vi "from string array.vi"(8 "error in (no error)":errorcluster, 9 "String Array":string[][](array[string]), 10 "version":string, 11 "PID Module configuration in":refnum<class "PID Module configuration.lvclass">) -> (0 "error out":errorcluster, 3 "PID Module configuration out":refnum<class "PID Module configuration.lvclass">)   [LabVIEW 2015, in "PID Module configuration.lvclass"]
uses:
  PID Module configuration.lvclass
  PID Module configuration.lvclass/PID Module configuration.ctl
  Write Lines.vi
  Get Line Name.vi
  <vilib>/NI/Tag Bus Module Framework/module configuration/FindDuplicate.vi
  <vilib>/Utility/error.llb/Error Cluster From Error Code.vi
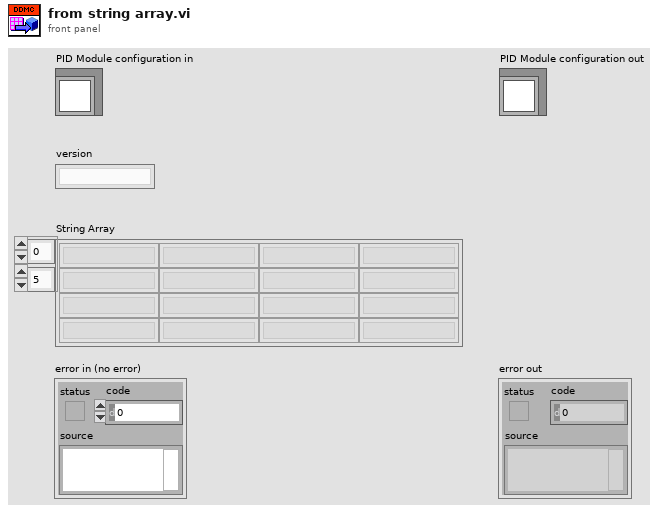
[diagram p1: front panel]
types:
  T1 = typedef "PID Module configuration.lvclass/Line.ctl" = cluster{"PID ID":string, "Setpoint":refnum<class "TBM channel.lvclass">, "Variable":refnum<class "TBM channel.lvclass">, "Output":refnum<class "TBM channel.lvclass">, "Output High":refnum<class "TBM channel.lvclass">, "Output Low":refnum<class "TBM channel.lvclass">, "P":refnum<class "TBM channel.lvclass">, "I":refnum<class "TBM channel.lvclass">, "D":refnum<class "TBM channel.lvclass">}
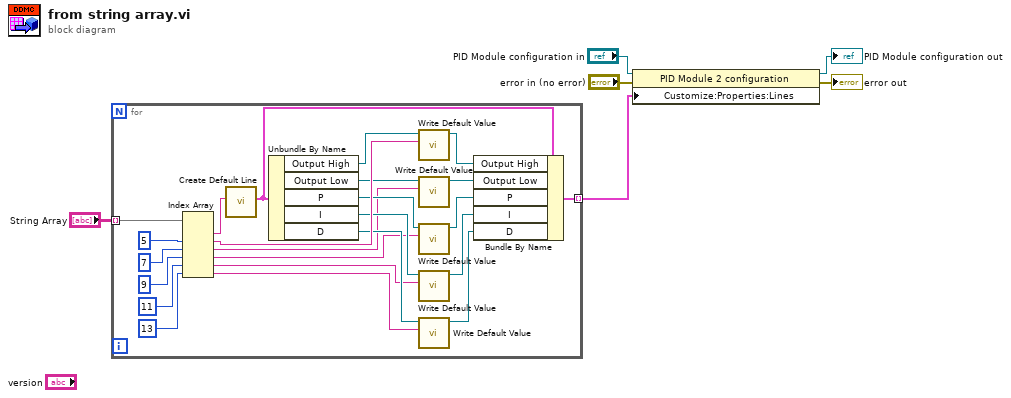
[diagram p0: block diagram]
diagram:
  n1 = for {
    tunnel: "String Array" -> [w30] mode=indexing
    tunnel: [w29] -> w1 mode=indexing
    n2 = Index Array(array=w30, index #2=5 ("index"), index #3=7 ("index"), index #4=9 ("index"), index #5=11 ("index"), index #6=13 ("index")) -> (element #1=w28:string, element #2=w24:string, element #3=w14:string, element #4=w13:string, element #5=w12:string, element #6=w11:string)  [unwired: 1 in]
    n3 = call "Create Default Line.vi"("Line Name"=w28) -> ("Default Line"=w27:T1)  [unwired: 10 in]
    n4 = Unbundle By Name(w27) -> ("Output High"=w25:refnum<class "TBM channel.lvclass">, "Output Low"=w20:refnum<class "TBM channel.lvclass">, "P"=w21:refnum<class "TBM channel.lvclass">, "I"=w22:refnum<class "TBM channel.lvclass">, "D"=w23:refnum<class "TBM channel.lvclass">)
    n5 = call "Write Default Value.vi"("Data"=w24, "Channel in"=w25) -> ("Channel out"=w26:refnum<class "TBM channel.lvclass">)  [unwired: 9 in]
    n6 = call "Write Default Value.vi"("Data"=w14, "Channel in"=w20) -> ("Channel out"=w19:refnum<class "TBM channel.lvclass">)  [unwired: 9 in]
    n7 = call "Write Default Value.vi"("Data"=w13, "Channel in"=w21) -> ("Channel out"=w18:refnum<class "TBM channel.lvclass">)  [unwired: 9 in]
    n8 = call "Write Default Value.vi"("Data"=w12, "Channel in"=w22) -> ("Channel out"=w17:refnum<class "TBM channel.lvclass">)  [unwired: 9 in]
    n9 = call "Write Default Value.vi"("Data"=w11, "Channel in"=w23) -> ("Channel out"=w16:refnum<class "TBM channel.lvclass">)  [unwired: 9 in]
    n10 = Bundle By Name(cluster=w27, "Output High"=w26, "Output Low"=w19, "P"=w18, "I"=w17, "D"=w16) -> (w29:T1)
  }
  n11 = property class="PID Module 2 configuration"(reference="PID Module configuration in", error in="error in (no error)", "Customize:Properties:Lines"=w1) -> (reference out=→"PID Module configuration out":refnum<class "PID Module configuration.lvclass">, error out=→"error out":errorcluster)
